vi "Array of String_Write Index Set.vi"(9 "Values":cluster{"String Array":string[]}[](array[cluster]), 11 "Indices":i32[](array[numeric])) -> ()   [LabVIEW 2016, in "CVT.lvlib" / "Current Value Table.lvlib"]
doc: "This VI writes a set of data as defined by the GetIndices function. This VI can provide an order of magnitude increase in performance over a normal index write for sufficiently large data sets."
uses:
  <vilib>/NI/Current Value Table/Current Value Table.lvlib
  <vilib>/NI/Current Value Table/Type Defs/Memory Commands.ctl
  <vilib>/NI/Current Value Table/DataTypes/Array of String_Memory Block.vi
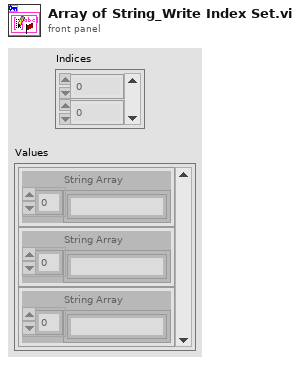
[diagram p1: front panel]
types:
  T1 = typedef "CVT.lvlib/Current Value Table.lvlib/Memory Commands.ctl" = enum16{"Init", "Add Data", "Read", "Read Group", "Read All", "Write", "Write Group", "Get Size"}
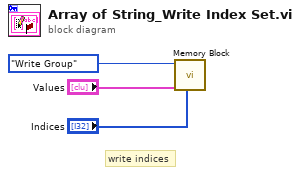
[diagram p0: block diagram]
diagram:
  # "write indices"
  n1 = call-poly <vilib>:"Memory Block.vi"("Group Indices"="Indices", "Data In"="Values", "Method"=Memory_Commands."Write Group") -> ()  [unwired: 6 in, 3 out]
